vi "Create Channel.vi"(6 "index":i32, 8 "error in":errorcluster, 10 "channel settings":T1, 11 "counter input pwm mode in":refnum<class "Counter Input PWM Mode.lvclass">) -> (0 "error out":errorcluster, 2 "channel out":refnum<class "PWM Input Channel.lvclass">, 3 "counter input pwm mode out":refnum<class "Counter Input PWM Mode.lvclass">)   [LabVIEW 2017, in "Scan Engine Scripting.lvlib" / "Counter Input PWM Mode.lvclass"]
doc: "Creates an instance of a channel."
uses:
  Counter Input PWM Mode.lvclass
  Controls/counter input pwm channel settings.ctl
  Channel Classes/PWM Input Channel/Measurement Type.ctl
  Channel Classes/PWM Input Channel/PWM Input Channel.lvclass
  Counter Input PWM Mode.lvclass/Counter Input PWM Mode.ctl
  Scan Engine Scripting.lvlib
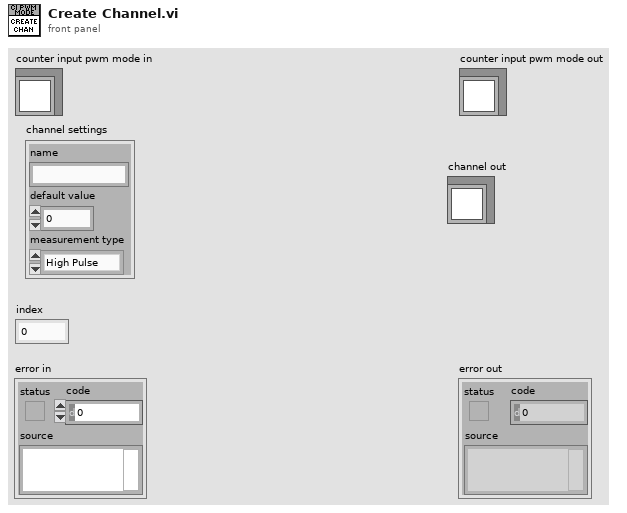
[diagram p1: front panel]
types:
  T1 = typedef "Scan Engine Scripting.lvlib/counter input pwm channel settings.ctl" = cluster{"name":string, "default value":dbl, "measurement type":T2}
  T2 = typedef "Scan Engine Scripting.lvlib/PWM Input Channel.lvclass/Measurement Type.ctl" = enum16{"High Pulse", "Low Pulse", "Most Recent"}
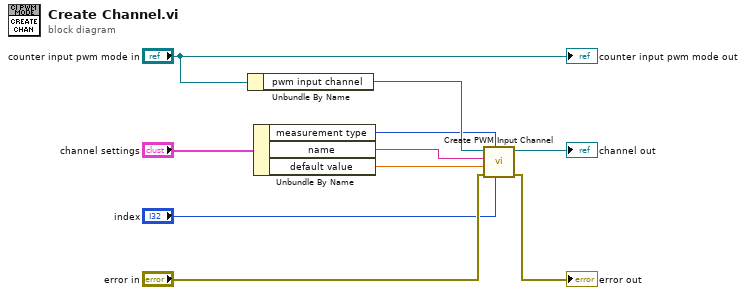
[diagram p0: block diagram]
diagram:
  n1 = Unbundle By Name("counter input pwm mode in") -> ("pwm input channel"=w7:refnum<class "PWM Input Channel.lvclass">)
  n2 = Unbundle By Name("channel settings") -> ("measurement type"=w4:T2, "name"=w3:string, "default value"=w2:dbl)
  n3 = call "Create PWM Input Channel.vi"("index"="index", "measurement type"=w4, "error in"="error in", "default value"=w2, "name"=w3, "PWM Input Channel.lvclass"=w7) -> ("error out"=→"error out":errorcluster, "channel out"=→"channel out":refnum<class "PWM Input Channel.lvclass">)  [unwired: 4 in]
  "counter input pwm mode out" <- "counter input pwm mode in"
